vi "Configure Dead Band And Travel Time.vi"(0 "VISA resource name":refnum<visa-resource-name>, 1 "Unit Address (1)":u8=1 min=1 max=254, 5 "Deadband (0)":sgl min=0 max=100 format="%.2g", 9 "Travel Time (0)":sgl min=0 max=1000 format="%.1g", 11 "error in (no error)":errorcluster) -> (4 "VISA resource name out":refnum<visa-resource-name>, 15 "error out":errorcluster)   [LabVIEW 2010, in "Eurotherm 32xx Series.lvlib"]
doc: "This VI sets Output Parameters."
uses:
  <instrlib>/Eurotherm 32xx Series/Eurotherm 32xx Series.lvlib
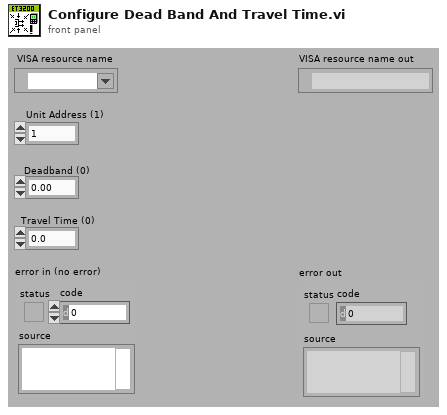
[diagram p1: front panel]
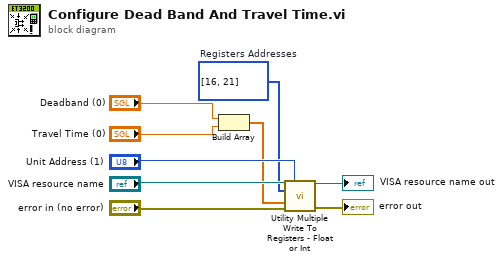
[diagram p0: block diagram]
diagram:
  w3 = u16[] [16, 21]  # Registers Addresses
  n1 = Build Array("Deadband (0)", "Travel Time (0)") -> (w4:sgl[])
  n2 = call <instrlib>:"Utility Multiple Write To Registers - Float or Int.vi"("VISA resource name"="VISA resource name", "Unit Address (1)"="Unit Address (1)", "Registers Addresses (0)"=w3, "Data (0)"=w4, "error in (no error)"="error in (no error)") -> ("VISA resource name out"=→"VISA resource name out":refnum<visa-resource-name>, "error out"=→"error out":errorcluster)  [unwired: 9 in]
